vi "Handle Command.vi"(8 "error in":errorcluster, 10 "CMD In":refnum<class "Change Speaker Vparams.lvclass">, 11 "Object In":refnum<class>) -> (0 "error out":errorcluster, 1 "Command Successful?":bool, 2 "CMD Out":refnum<class "Change Speaker Vparams.lvclass">, 3 "Object Out":refnum<class>)   [LabVIEW 2014, in "ePAS Library.lvlib" / "Change Speaker Vparams.lvclass"]
doc: "Abstract method for accomplishing the execution of a command directed to an instrument object on the wire."
uses:
  Change Speaker Vparams.lvclass
  Instrument/ePAS.lvclass
  Instrument/ePAS.lvclass/ePAS.ctl
  reusable/Instrument/Instrument.lvclass/Instrument.ctl
  Change Speaker Vparams.lvclass/Change Speaker Vparams.ctl
  Instrument/Accessors/Read FPGA Session.vi
  reusable/Instrument/Read Log Session.vi
  <vilib>/Utility/error.llb/Error Cluster From Error Code.vi
  <vilib>/rvi/errors/niLvFpgaAdjustHostInterfaceError.vi
  <userlib>/_Session Fwk/Session - Root.lvclass
  <vilib>/rvi/interface/nirviReadWriteControl/nirviReadWriteControl.xnode
  FPGA/R FPGA Ref.ctl
  FPGA Bitfiles/FPGA Server.lvbitx
  FPGA/Session/Exscalabar FPGA.lvclass
  ePAS Library.lvlib
  reusable/Session APIs/Session Log/System Log.lvclass
  NiFpgaLv.dll
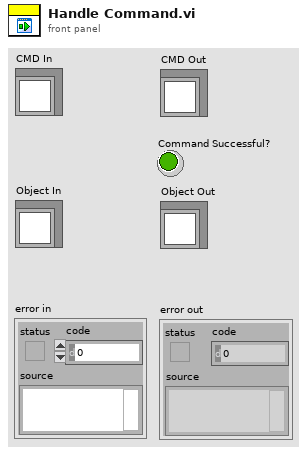
[diagram p1: front panel]
types:
  T1 = typedef "Session - Root.lvclass/Session Handle.ctl" = refnum<data-value>
  T2 = typedef "ePAS Library.lvlib/R FPGA Ref.ctl" = refnum<k20>
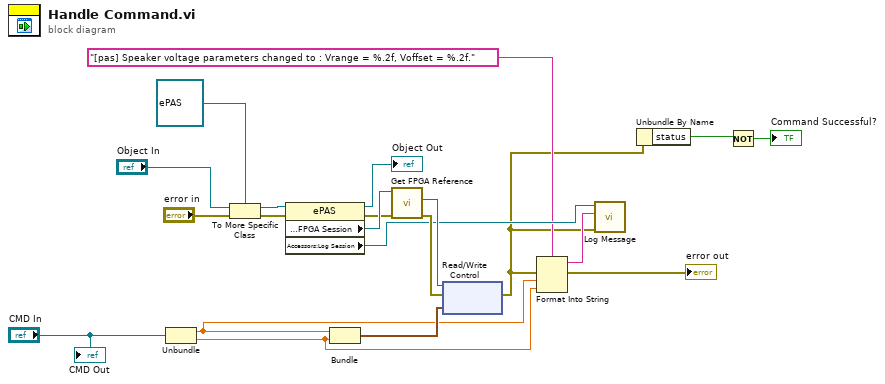
[diagram p0: block diagram]
diagram:
  n1 = Unbundle("CMD In") -> (w6:dbl, w5:dbl)
  n2 = To More Specific Class(target class=refnum<class "ePAS.lvclass"> refnum ("ePAS"), reference="Object In", error in="error in") -> (specific class reference=w20:refnum<class "ePAS.lvclass">, error out=w21:errorcluster)
  n3 = property class="ePAS"(reference=w20, error in=w21) -> (reference out=→"Object Out":refnum<class "ePAS.lvclass">, error out=w17:errorcluster, "Accessors:FPGA Session"=w18:T1, "Accessors:Log Session"=w13:T1)
  n4 = Bundle("Vrange"=w6, "Voffset"=w5) -> (w7:cluster{"Vrange":dbl, "Voffset":dbl})  [unwired: 1 in]
  n5 = call "Get FPGA Reference.vi"("error in"=w17, "Session In"=w18) -> ("error out"=w14:errorcluster, "Ex FPGA Ref"=w15:T2)  [unwired: 7 in, 1 out]
  n6 = xnode "Read/Write Control"("FPGA VI Reference In"=w15, "error in"=w14, "Speaker"=w7) -> ("error out"=w4:errorcluster)  [unwired: 1 out]
  n7 = Format Into String(format string="[pas] Speaker voltage parameters changed to : Vrange = %.2f, Voffset = %.2f.", error in=w4, w6, w5) -> (resulting string=w11:string, error out=→"error out":errorcluster)  [unwired: 1 in]
  n8 = call "Log Message.vi"("error in"=w4, "MSG In"=w11, "session in"=w13) -> ()  [unwired: 7 in, 2 out]
  n9 = Unbundle By Name(w4) -> ("status"=w3:bool)
  n10 = Not(x=w3) -> (.not. x?=→"Command Successful?":bool)
  "CMD Out" <- "CMD In"
